vi "dfd_Nyquist Design with Order.vi"(4 "fs in [Hz]":dbl=1.0 format="%#_2g", 5 "method":u16(ring)=3 items=["Kaiser Window", "Dolph-Chebyshev Window", "Equi-Ripple", "Positive Equi-Ripple"], 6 "filtering mode":T1=2 items=["No Rate Change", "Interpolation", "Decimation"], 7 "multirate factor":i32=4, 8 "error in (no error)":errorcluster, 10 "roll off":dbl=0.2, 11 "order":i32=10) -> (0 "error out":errorcluster, 2 "order out":i32, 3 "multirate filter out":T2={"mMRate_Structure"=enum."FIR", "mMRate_Mode"=0, "mMRate_Factor"=4, "mMRate_FIRParams"={"mMRate_FIR_H"=[2.3609188004286374e-07, 6.198015209266301e-07, 5.848786504097344e-07, 0.0, -1.3686726929583832e-06, -2.650607020100775e-06, -2.5718438519774773e-06, 0.0, 4.54297851657941e-06, 8.385553691280157e-06, 7.63647912970769e-06, 0.0, -1.2279335303775897e-05, -2.171206376084249e-05, -1.9039675696856382e-05, 0.0, 2.8639896742556653e-05, 4.9181414551547944e-05, 4.197195097043475e-05, 0.0, -6.0122545671642824e-05, -0.0001009805959862553, -8.439921959047963e-05, 0.0, 0.0001163549293011043, 0.00019200870840356966, 0.00015781185965919056, 0.0, -0.00021088599514298276, -0.0003429848254355214, -0.0002780106524137319, 0.0, 0.0003619608265250965, 0.0005815418773280012, 0.000465878287089251, 0.0, -0.000593300220473181, -0.0009433469242277491, -0.0007481929202042657, 0.0, 0.0009349946056241044, 0.001473456855245187, 0.0011586739407478252, 0.0, -0.0014248106640678704, -0.002228431325834784, -0.001739711500903688, 0.0, 0.0021105765428306583, 0.0032803357988940014, 0.002545742267607504, 0.0, -0.003055036507256795, -0.004725008184504415, -0.0036503035326915546, 0.0, 0.004346186536858871, 0.00669980952177101, 0.005161314707831401, 0.0, -0.006120138844470059, -0.009423405331132886, -0.0072558463037462545, 0.0, 0.008615147114073421, 0.013291971310205309, 0.010266465802877451, 0.0, -0.012314710100654363, -0.0191441135833648, -0.014929688022798955, 0.0, 0.018405529850789665, 0.029165173024403242, 0.0232993269907664, 0.0, -0.03080739883635062, -0.05141057805520357, -0.04404451287832945, 0.0, 0.07443979508119634, 0.1586007825160465, 0.22488286686884343, 0.25000022035892416, 0.22488286686884343, 0.1586007825160465, 0.07443979508119634, 0.0, -0.04404451287832945, -0.05141057805520357, -0.03080739883635062, 0.0, 0.0232993269907664, 0.029165173024403242, 0.018405529850789665, 0.0, -0.014929688022798955, -0.0191441135833648, -0.012314710100654363, 0.0, 0.010266465802877451, 0.013291971310205309, 0.008615147114073421, 0.0, -0.0072558463037462545, -0.009423405331132886, -0.006120138844470059, 0.0, 0.005161314707831401, 0.00669980952177101, 0.004346186536858871, 0.0, -0.0036503035326915546, -0.004725008184504415, -0.003055036507256795, 0.0, 0.002545742267607504, 0.0032803357988940014, 0.0021105765428306583, 0.0, -0.001739711500903688, -0.002228431325834784, -0.0014248106640678704, 0.0, 0.0011586739407478252, 0.001473456855245187, 0.0009349946056241044, 0.0, -0.0007481929202042657, -0.0009433469242277491, -0.000593300220473181, 0.0, 0.000465878287089251, 0.0005815418773280012, 0.0003619608265250965, 0.0, -0.0002780106524137319, -0.0003429848254355214, -0.00021088599514298276, 0.0, 0.00015781185965919056, 0.00019200870840356966, 0.0001163549293011043, 0.0, -8.439921959047963e-05, -0.0001009805959862553, -6.0122545671642824e-05, 0.0, 4.197195097043475e-05, 4.9181414551547944e-05, 2.8639896742556657e-05, 0.0, -1.9039675696856382e-05, -2.1712063760842487e-05, -1.2279335303775897e-05, 0.0, 7.63647912970769e-06, 8.385553691280157e-06, 4.54297851657941e-06, 0.0, -2.5718438519774773e-06, -2.650607020100775e-06, -1.3686726929583813e-06, 0.0, 5.848786504097363e-07, 6.198015209266313e-07, 2.3609188004286673e-07], "mMRate_FIR_IsNyquist?"=FALSE, "mMRate_FIR_IsSymmetric?"=FALSE}, "mMRate_CICParams"={"mMRate_CIC_#Stage"=2, "mMRate_CIC_Lag"=1, "mMRate_CIC_Type"=enum."Lowpass"}, "mMRate_Order"=166, "mMRate_Version"="1.0", "mMRate_Comments"="1.0", "mMRate_RationalFactor"={"mMRate_L"=-1, "mMRate_M"=-1}, "mMRate_Fs"=1.0, "mMRate_Quantized?"=FALSE, "mMRate_QFilterGain"=1.0, "mMRate_CoefWl"=16, "mMRate_Scaling"={"mMRate_ScaleByPowerOf2?"=FALSE, "mMRate_ScaleType"=enum."Time Domain 1-Norm"}, "mMRate_InputWl"=0, "mMRate_OutputWl"=0, "mMRate_OutputMode"=enum."Nearest", "mMRate_MultMode"=enum."Truncated", "mMRate_BitPruning"=FALSE, "mMRate_GainWl"=16, "mMRate_OutputFwl"=0, "mMRate_SumIwl"=0, "mMRate_InputIwl "=16, "mMRate_SumWl"=32, "mMRate_CoefIwl"=0} {"mMRate_SumWl" min=1 max=32 step=1; "mMRate_InputIwl" min=1 max=32 step=1; "mMRate_GainWl" min=1 max=32 step=1; "mMRate_OutputWl" min=1 max=32 step=1; "mMRate_InputWl" min=1 max=32 step=1; "mMRate_CoefWl" min=1 max=32 step=1; "mMRate_Mode" items=["Default"=-1, "No Rate Change"=0, "Interpolation"=1, "Decimation"=2, "Interpolated"=3, "Rational"=4]})   [LabVIEW 2017, in "NI_DigFilterLicensed.lvlib"]
doc: "Designs a Nyquist filter with order specified. The filter can be used as a normal filter, an interpolator or a decimator."
uses:
  <vilib>/addons/Digital Filter Design/NI_DigFilterLicensed.lvlib
  <vilib>/addons/Digital Filter Design/_Objects.llb/DFD Multirate Filter Obj.ctl
  <vilib>/addons/Digital Filter Design/_Objects.llb/DFD Multirate Mode.ctl
  <vilib>/addons/Digital Filter Design/_Objects.llb/DFD Coef Norm Type.ctl
  <vilib>/addons/Digital Filter Design/_Objects.llb/DFD Round-off Mode.ctl
  <vilib>/addons/Digital Filter Design/_Objects.llb/DFD FXP MRate Multiply Mode.ctl
  <vilib>/addons/Digital Filter Design/_Objects.llb/DFD Multirate Filtering Mode.ctl
  <vilib>/addons/Digital Filter Design/FilterLib.llb/DFD Build MRate Filter from TF.vi
  <vilib>/addons/Digital Filter Design/NI_DigFilter_Process.lvlib
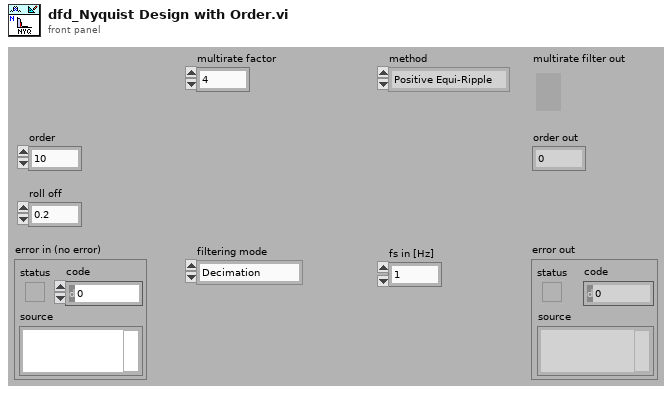
[diagram p1: front panel]
types:
  T1 = typedef "NI_DigFilterLicensed.lvlib/DFD Multirate Filtering Mode.ctl" = u16
  T2 = typedef "NI_DigFilterLicensed.lvlib/DFD Multirate Filter Obj.ctl" = cluster{"mMRate_Structure":enum16{"CIC", "FIR", "IIR", "Lattice"}, "mMRate_Mode":T3, "mMRate_Factor":i32, "mMRate_FIRParams":cluster{"mMRate_FIR_H":dbl[], "mMRate_FIR_IsNyquist?":bool, "mMRate_FIR_IsSymmetric?":bool}, "mMRate_CICParams":cluster{"mMRate_CIC_#Stage":i32, "mMRate_CIC_Lag":i32, "mMRate_CIC_Type":enum16{"Lowpass", "Highpass"}}, "mMRate_Order":i32, "mMRate_Version":string, "mMRate_Comments":string, "mMRate_RationalFactor":cluster{"mMRate_L":i32, "mMRate_M":i32}, "mMRate_Fs":dbl, "mMRate_Quantized?":bool, "mMRate_QFilterGain":dbl, "mMRate_CoefWl":i16, "mMRate_Scaling":cluster{"mMRate_ScaleByPowerOf2?":bool, "mMRate_ScaleType":T4}, "mMRate_InputWl":i16, "mMRate_OutputWl":i16, "mMRate_OutputMode":T5, "mMRate_MultMode":T6, "mMRate_BitPruning":bool, "mMRate_GainWl":i16, "mMRate_OutputFwl":i16, "mMRate_SumIwl":i16, "mMRate_InputIwl ":i16, "mMRate_SumWl":i16, "mMRate_CoefIwl":i16}
  T3 = typedef "NI_DigFilterLicensed.lvlib/DFD Multirate Mode.ctl" = i16
  T4 = typedef "NI_DigFilterLicensed.lvlib/DFD Coef Norm Type.ctl" = enum16{"No Norm", "Time Domain 1-Norm", "Time Domain 2-Norm", "Time Domain Inf-Norm"}
  T5 = typedef "NI_DigFilterLicensed.lvlib/DFD Round-off Mode.ctl" = enum16{"Nearest", "Truncation"}
  T6 = typedef "NI_DigFilterLicensed.lvlib/DFD FXP MRate Multiply Mode.ctl" = enum16{"Truncated", "Full"}
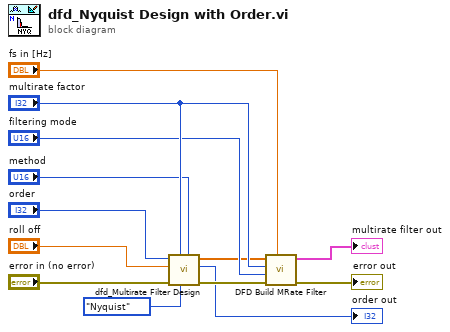
[diagram p0: block diagram]
diagram:
  n1 = call <vilib>:"dfd_Multirate Filter Design.vi"("method"="method", "band option"=enum16{"Normal", "Nyquist", "Alias free"}."Nyquist", "#band"="multirate factor", "error IO"="error in (no error)", "roll off"="roll off", "order"="order") -> ("error out"=w6:errorcluster, "order out"=→"order out":i32, "h out"=w7:dbl[])  [unwired: 3 in]
  n2 = call-poly <vilib>:"DFD Build MRate Filter.vi"("fs in [Hz]"="fs in [Hz]", "error in (no error)"=w6, "filtering mode"="filtering mode", "factor"="multirate factor", "h(n)"=w7) -> ("error out"=→"error out":errorcluster, "multirate filter out"=→"multirate filter out":T2)  [unwired: 5 out]
